vi "write_fifo.vi"(7 "pixel-to-host\n mode":T1, 8 "FIFO overflow in":bool, 9 "maximum bit depth":i8, 10 "block index in":i32, 11 "values to be written":T2) -> (0 "FIFO overflow out":bool, 2 "block index out":i32, 3 "channels out":T2)   [LabVIEW 2010]
uses:
  common_typedefs/channels_cluster.ctl
  common_typedefs/pixel_to_host_enum.ctl
  <vilib>/rvi/DataTransferAndStorage/Container/XNode/niFpgaContainer.xnode
  <vilib>/rvi/DataTransferAndStorage/Container/Common/niFpgaContainerMethod.ctl
  <vilib>/rvi/DataTransferAndStorage/Container/Common/niFpgaTransferTypeControl.ctl
  <vilib>/rvi/interface/RandomDataEmulation/nirviRandomDataFPGAFIFO.vi
  <vilib>/rvi/interface/RandomDataEmulation/niFpgaRandomDataHandleErrors.vi
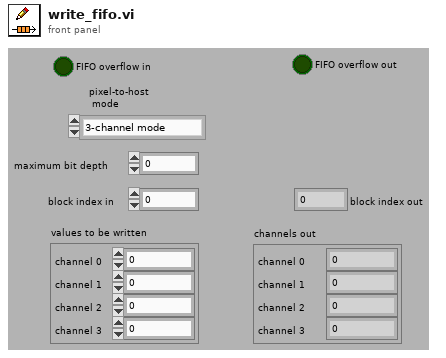
[diagram p1: front panel]
types:
  T1 = typedef "pixel_to_host_enum.ctl" = enum16{"3-channel mode", "4-channel mode"}
  T2 = typedef "channels_cluster.ctl" = cluster{"channel 0":u32, "channel 1":u32, "channel 2":u32, "channel 3":u32}
  T3 = typedef "niFpgaContainerMethod.ctl" = enum16{"<none>", "write", "read", "clear", "getNumberOfElementsToWrite", "getNumberOfElementsToRead", "enable", "disable", "flushAndDisable", "getStreamState", "readA", "readB", "dramWrite", "dramWriteWithByteEnables", "dramRequestData", "dramRetrieveData"}
  T4 = typedef "niFpgaTransferTypeControl.ctl" = enum16{"Target-Scoped", "Host to Target - DMA", "Target to Host - DMA", "Peer to Peer Reader", "Peer to Peer Writer", "Bidirectional"}
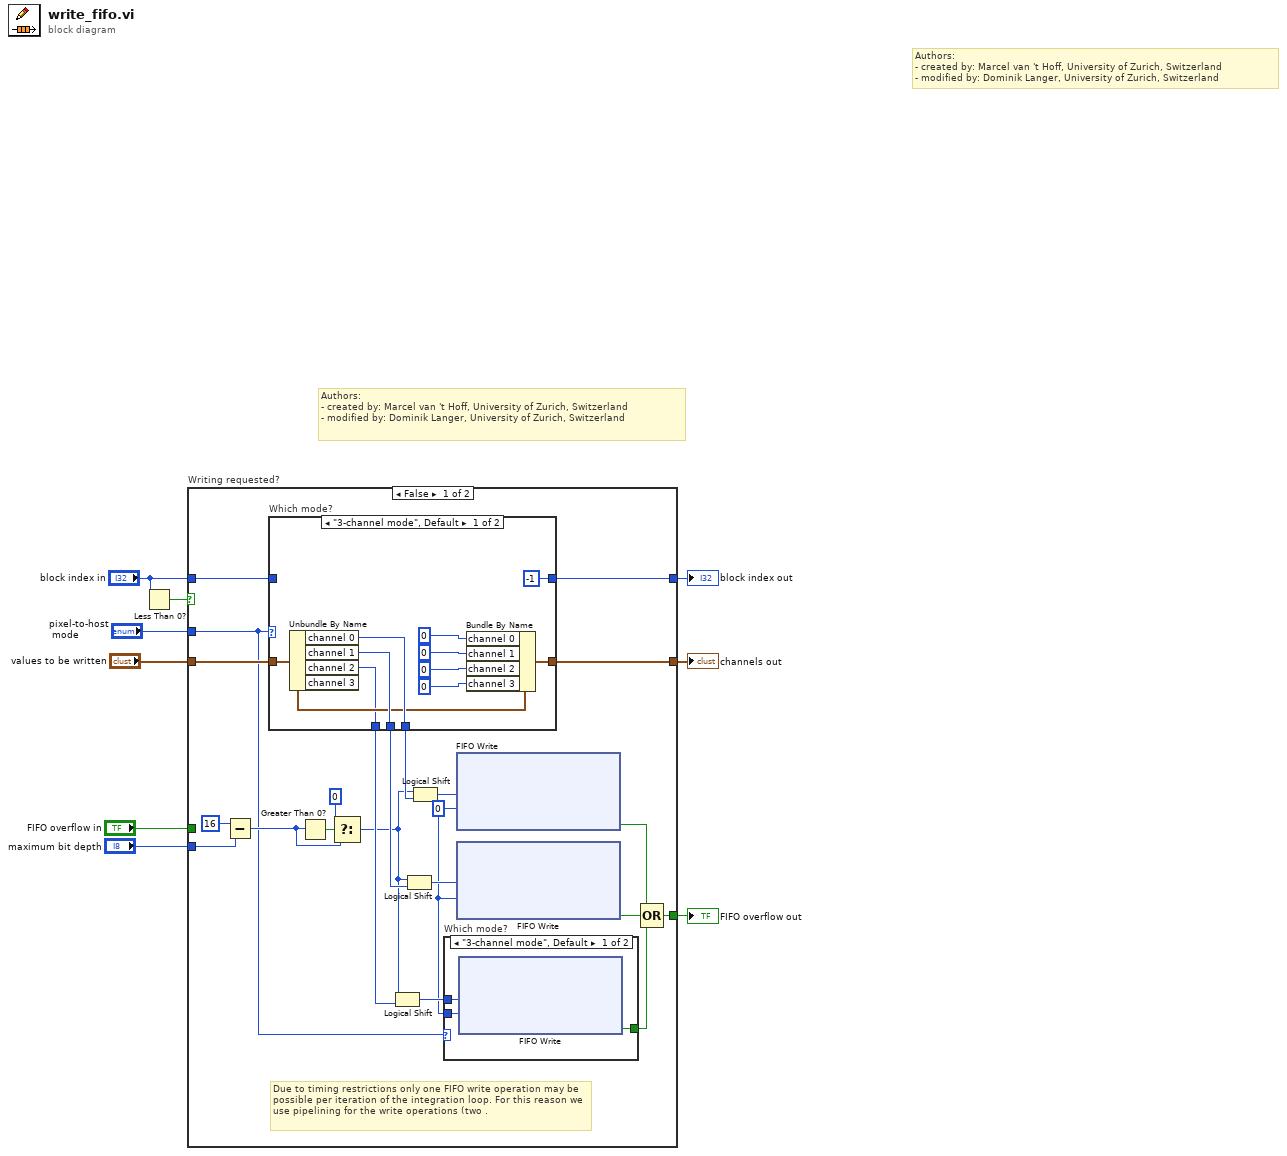
[diagram p0: block diagram]
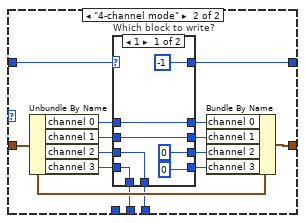
[diagram p3: hidden frame]
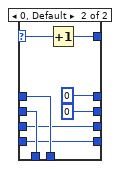
[diagram p4: hidden frame]
diagram:
  # "Authors: \n- created by: Marcel van 't Hoff, University of Zurich, Switzerland\n- modified by: Dominik Langer, University of Zurich, Switzerland"
  # "Authors: \n- created by: Marcel van 't Hoff, University of Zurich, Switzerland\n- modified by: Dominik Langer, University of Zurich, Switzerland"
  n1 = Less Than 0?(x="block index in") -> (x < 0?=w4:bool)
  n2 = case "Writing requested?" shown="False" w4 {
    tunnel: [w23 w159] -> w5
    tunnel: [w20 w160] -> w9
    tunnel: "maximum bit depth" -> [w27 _]
    tunnel: "block index in" -> [w22 w160]
    tunnel: "values to be written" -> [w21 w159]
    tunnel: "FIFO overflow in" -> [_ w158]
    tunnel: [w24 w158] -> w2
    tunnel: "pixel-to-host\n mode" -> [w12 _]
    frame False {
      w10 = 0 ("Timeout")
      # "Due to timing restrictions only one FIFO write operation may be possible per iteration of the integration loop. For this reason we use pipelining for the write operations (two ."
      n3 = Subtract(x=i8 16, y=w27) -> (x-y=w29:i8)
      n4 = case "Which mode?" shown="\"3-channel mode\", Default" w12 {
        tunnel: [w66 w76] -> w23
        tunnel: w22 -> [_ w73]
        tunnel: w21 -> [w65 w78]
        tunnel: [-1 ("block index in") w77] -> w20
        tunnel: [w71 w75] -> w19
        tunnel: [w72 w74] -> w18
        tunnel: [w63 _] -> w14
        frame "3-channel mode", Default {
          n5 = Unbundle By Name(w65) -> ("channel 0"=w72:u32, "channel 1"=w71:u32, "channel 2"=w63:u32)  [unwired: 1 out]
          n6 = Bundle By Name(cluster=w65, "channel 0"=u32 0, "channel 1"=u32 0, "channel 2"=u32 0 ("channel 0"), "channel 3"=u32 0 ("channel 1")) -> (w66:T2)
        }
        frame "4-channel mode" {
          n7 = Unbundle By Name(w78) -> ("channel 0"=w79:u32, "channel 1"=w80:u32, "channel 2"=w81:u32, "channel 3"=w82:u32)
          n8 = case "Which block to write?" shown="1" w73 {
            selector: w73 -> [_ w94]
            tunnel: [w93 w101] -> w74
            tunnel: w79 -> [w91 w101]
            tunnel: [w92 w100] -> w75
            tunnel: w80 -> [w90 w100]
            tunnel: w81 -> [w93 w99]
            tunnel: w82 -> [w92 w98]
            tunnel: [u32 0 ("channel 2") w99] -> w84
            tunnel: [u32 0 ("channel 3") w98] -> w83
            tunnel: [w91 u32 0 ("channel 0")] -> w85
            tunnel: [w90 u32 0 ("channel 1")] -> w86
            tunnel: [-1 ("block index in") w95] -> w77
            frame 1 {
            }
            frame 0, Default {
              n9 = Increment(x=w94) -> (x+1=w95:i32)
            }
          }
          n10 = Bundle By Name(cluster=w78, "channel 0"=w85, "channel 1"=w86, "channel 2"=w84, "channel 3"=w83) -> (w76:T2)
        }
      }
      n11 = Greater Than 0?(x=w29) -> (x > 0?=w28:bool)
      n12 = Select(t=i8 0 ("f"), s=w28, f=w29) -> (s? t:f=w13:i8)
      n13 = Logical Shift(y=w13, x=w14) -> (x << y=w11:u32)
      n14 = Logical Shift(y=w13, x=w19) -> (x << y=w17:u32)
      n15 = Logical Shift(y=w13, x=w18) -> (x << y=w16:u32)
      n16 = case "Which mode?" shown="\"3-channel mode\", Default" w12 {
        tunnel: [w34 _] -> w15
        tunnel: w11 -> [w33 _]
        tunnel: w10 -> [w32 _]
        frame "3-channel mode", Default {
          n17 = xnode ("FIFO Write")("Element"=w33, "Timeout"=w32) -> ("Timed Out?"=w34:bool)  [unwired: 1 in, 1 out]
        }
        frame "4-channel mode" {
        }
      }
      n18 = xnode ("FIFO Write")("Element"=w16, "Timeout"=w10) -> ("Timed Out?"=w25:bool)  [unwired: 1 in, 1 out]
      n19 = xnode ("FIFO Write")("Element"=w17, "Timeout"=w10) -> ("Timed Out?"=w26:bool)  [unwired: 1 in, 1 out]
      n20 = Compound Arithmetic op=OR(w25, w26, w15) -> (w24:bool)
    }
    frame True {
    }
  }
  "channels out" <- w5
  "block index out" <- w9
  "FIFO overflow out" <- w2
